vi "FTW-ZMQ-LibraryFilepath.vi"(11 "error in":errorcluster) -> (4 "FTW-ZMQ Library Filepath":path, 6 "ZMQ Version":string, 15 "error out":errorcluster)   [LabVIEW 2012, in "FTW-ZMQ-Context.lvclass"]
uses:
  Context/FTW-ZMQ-Context.lvclass
panel:
  # "Inputs"
  # "Outputs"
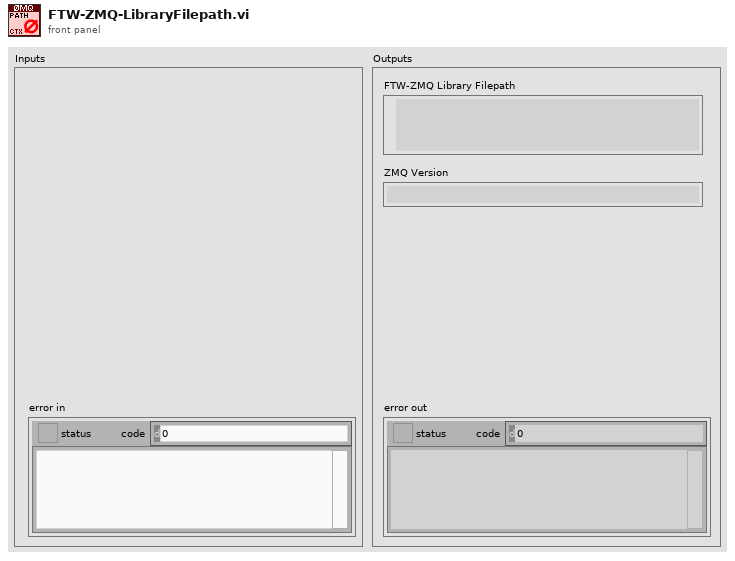
[diagram p1: front panel]
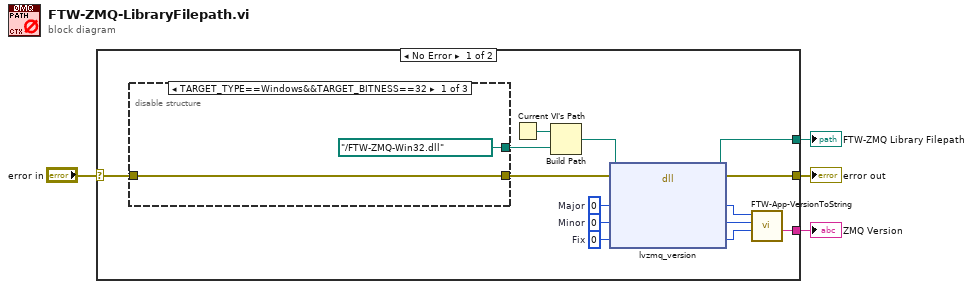
[diagram p0: block diagram]
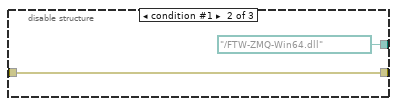
[diagram p2: hidden frame]
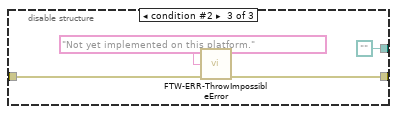
[diagram p3: hidden frame]
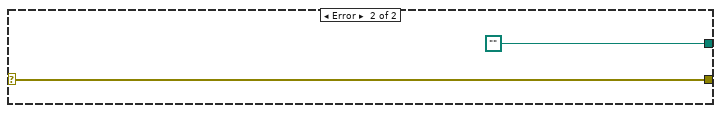
[diagram p4: hidden frame]
diagram:
  n1 = case shown="No Error" "error in" {
    selector: "error in" -> [w9 w28]
    tunnel: [w15 path ""] -> w4
    tunnel: [w13 w28] -> w3
    tunnel: [w5 _] -> w1
    frame No Error {
      w10 = 0  # Fix
      w11 = 0  # Minor
      w12 = 0  # Major
      n2 = disable-structure shown="TARGET_TYPE==Windows&&TARGET_BITNESS==32" {
        disable-tunnel: [path "../FTW-ZMQ-Win32.dll" path "../FTW-ZMQ-Win64.dll" path ""] -> w17
        disable-tunnel: [w20 w21 w25] -> w14
        disable-tunnel: w9 -> [w20 w21 w26]
        frame condition #0 (active) {
        }
        frame condition #1 {
        }
        frame condition #2 {
          n3 = call "FTW-ERR-ThrowImpossibleError.vi"("Reason this error should never happen"="Not yet implemented on this platform.", "error in"=w26) -> ("error out"=w25:errorcluster)  [unwired: 13 in]
        }
      }
      n4 = Current VI's Path() -> (path=w18:path)
      n5 = Build Path(base path=w18, name or relative path=w17) -> (appended path=w16:path)
      n6 = dll-call lib="?" fn="lvzmq_version" ("zmq_labview.dll:lvzmq_socket")(path in=w16, error in=w14, "Major"=w12, "Minor"=w11, "Fix"=w10) -> (path out=w15:path, error out=w13:errorcluster, "Major"=w8:i32, "Minor"=w7:i32, "Fix"=w6:i32)  [unwired: 2 in]
      n7 = call "FTW-App-VersionToString.vi"("Fix"=w6, "Minor"=w7, "Major"=w8) -> ("Version (minus Build)"=w5:string)  [unwired: 7 in, 1 out]
    }
    frame Error {
    }
  }
  "error out" <- w3
  "FTW-ZMQ Library Filepath" <- w4
  "ZMQ Version" <- w1
